vi "Gain Add or Remove.vi"(8 "error in (no error)":errorcluster, 9 "Name Prefix":string, 10 "Size":i32, 11 "Channel Gain":T1) -> (0 "error out":errorcluster, 3 "Channel Gain out":T1)   [LabVIEW 2019, in "Instrument.Lockin.lvlib" / "Instrument.DAQ.lvclass"]
uses:
  Instrument.DAQ.lvclass
  Typedefs/Channel.Gain--Cluster--Array.ctl
  Typedefs/Channel.Gain--Cluster.ctl
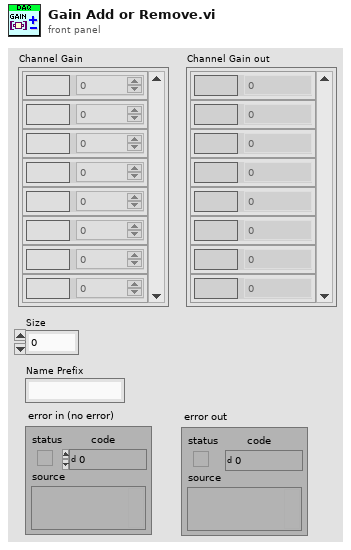
[diagram p1: front panel]
types:
  T1 = typedef "Instrument.Lockin.lvlib/Instrument.DAQ.lvclass/Channel.Gain--Cluster--Array.ctl" = T2[]
  T2 = typedef "Instrument.Lockin.lvlib/Instrument.DAQ.lvclass/Channel.Gain--Cluster.ctl" = cluster{"Channel":string, "Gain":dbl}
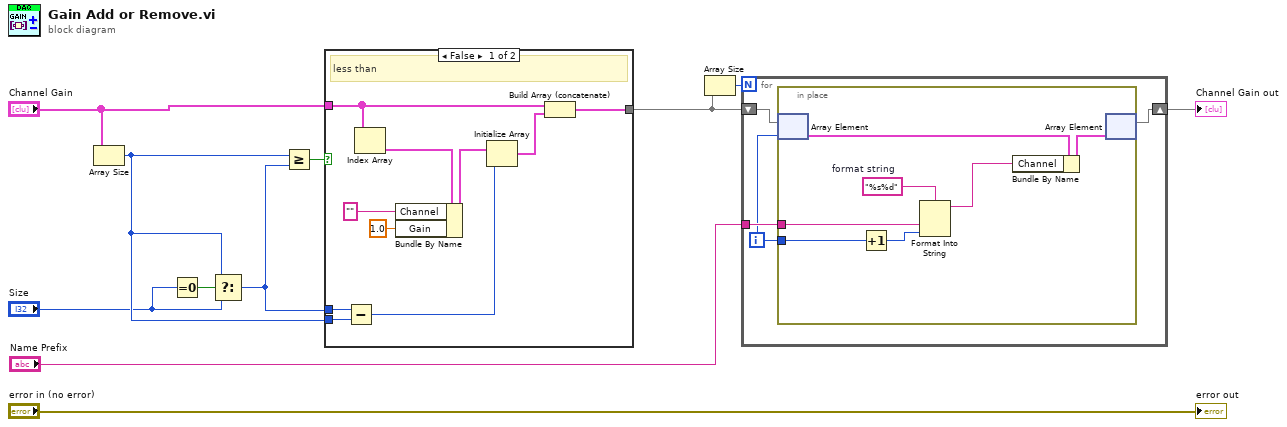
[diagram p0: block diagram]
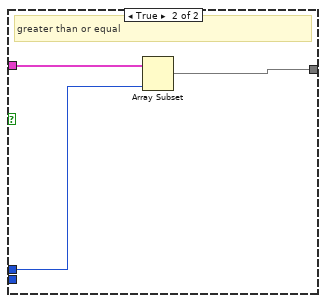
[diagram p2: hidden frame]
diagram:
  n1 = Array Size(array="Channel Gain") -> (size(s)=w3:i32)
  n2 = Equal To 0?(x="Size") -> (x = 0?=w4:bool)
  n3 = Select(t=w3, s=w4, f="Size") -> (s? t:f=w1:i32)
  n4 = Greater Or Equal?(x=w3, y=w1) -> (x >= y?=w5:bool)
  n5 = case shown="False" w5 {
    tunnel: "Channel Gain" -> [w15 w24]
    tunnel: w1 -> [w19 w23]
    tunnel: [w20 w22] -> w7
    tunnel: w3 -> [w18 _]
    frame False {
      # "less than"
      n6 = Subtract(x=w19, y=w18) -> (x-y=w17:i32)
      n7 = Index Array(array=w15) -> (element=w14:T2)  [unwired: 1 in]
      n8 = Bundle By Name(cluster=w14, "Channel"="", "Gain"=1.0) -> (w16:T2)
      n9 = Initialize Array(w16, w17) -> (w21:T2[])
      n10 = Build Array (concatenate)(w15, w21) -> (w20:T1)
    }
    frame True {
      # "greater than or equal"
      n11 = Array Subset(array=w24, length=w23) -> (w22:T1)  [unwired: 1 in]
    }
  }
  n12 = Array Size(array=w7) -> (size(s)=w8:i32)
  n13 = for {
    N: w8 -> [_]
    tunnel: "Name Prefix" -> [w28]
    shift-right: [w27] -> w11
    shift-left: w7 -> [w25]
    i -> [w26]
    n14 = in-place {
      in-place-border: w26 -> [w35]
      in-place-border: w28 -> [w32]
      w34 = "%s%d"  # format string
      n15 = in-place-array #1(w25, w26) -> (w31:T2)
      n16 = Increment(x=w35) -> (x+1=w33:i32)
      n17 = Format Into String(format string=w34, w32, w33) -> (resulting string=w29:string)  [unwired: 2 in, 1 out]
      n18 = Bundle By Name(cluster=w31, "Channel"=w29) -> (w30:T2)
      n19 = in-place-array #1(w30) -> (w27:T1)  [unwired: 1 out]
    }
  }
  "Channel Gain out" <- w11
  "error out" <- "error in (no error)"
